vi "Class Loading Progress.vi"(8 "error in (no error)":errorcluster, 10 "Progress (%)":T1 scale=0.0..100.0, 11 "Class Loader Interfaces in":refnum<class "Class Loader Interfaces.lvclass">) -> (0 "error out":errorcluster, 3 "Class Loader Interfaces out":refnum<class "Class Loader Interfaces.lvclass">)   [LabVIEW 2023, in "Class Loader Interfaces.lvlib" / "Class Loader Interfaces.lvclass"]
uses:
  Class Loader Interfaces.lvclass
  Class Loader/Loading Progress.ctl
  Class Loader/Class Loader.lvclass
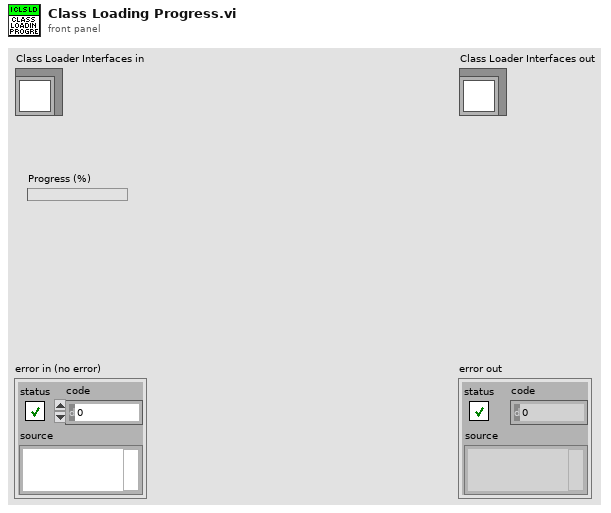
[diagram p1: front panel]
types:
  T1 = typedef "Class Loader.lvlib/Class Loader.lvclass/Loading Progress.ctl" = dbl
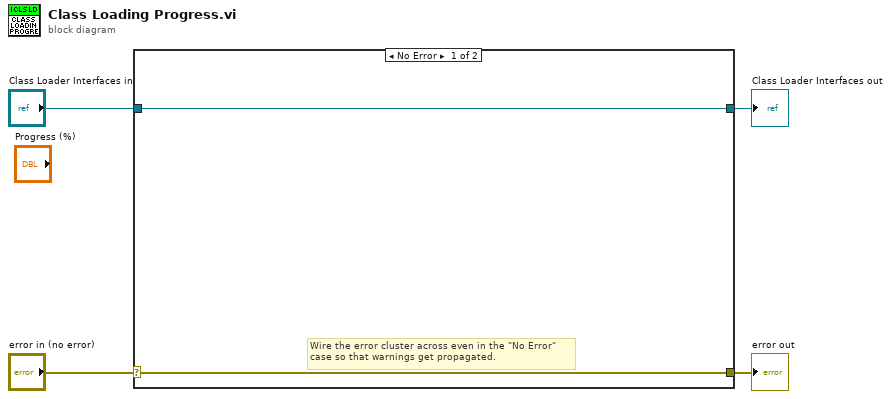
[diagram p0: block diagram]
diagram:
  n1 = case shown="No Error" "error in (no error)" {
    selector: "error in (no error)" -> [w5 w8]
    tunnel: [w5 w8] -> w3
    tunnel: [w6 w7] -> w1
    tunnel: "Class Loader Interfaces in" -> [w6 w7]
    frame No Error {
      # "Wire the error cluster across even in the \"No Error\"\ncase so that warnings get propagated."
    }
    frame Error {
    }
  }
  "error out" <- w3
  "Class Loader Interfaces out" <- w1
